vi "C400_module_SR.vi"() -> ()   [LabVIEW 2018]
panel:
  in  "autoconnect":bool=TRUE
  out "Ch1 Position Units":string
  out "Ch1Range":i32
  out "Ch1 Sensor Read":dbl format="%.3f"
  out "Serial Numbers":string[](array[string])
  out "FT_Status":u64(ring) items=["FT_OK", "FT_INVALID_HANDLE", "FT_DEVICE_NOT_FOUND", "FT_DEVICE_NOT_OPENED", "FT_IO_ERROR", "FT_INSUFFICIENT_RESOURCES", "FT_INVALID_PARAMETER", "FT_INVALID_BAUD_RATE", "FT_DEVICE_NOT_OPENED_FOR_ERASE", "FT_DEVICE_NOT_OPENED_FOR_WRITE", "FT_FAILED_TO_WRITE_DEVICE", "FT_EEPROM_READ_FAILED", "FT_EEPROM_WRITE_FAILED", "FT_EEPROM_ERASE_FAILED", "FT_EEPROM_NOT_PRESENT", "FT_EEPROM_NOT_PROGRAMMED", "FT_INVALID_ARGS", "FT_NOT_SUPPORTED", "FT_OTHER_ERROR"]
  in  "Ch1 Position Set":dbl step=50.0 format="%.3f"
  in  "Connect":bool
  in  "Stop VI":bool caption="Stop Button"
  in  "Found piezos":i32(listbox)=-1
  in  "Handle":u64
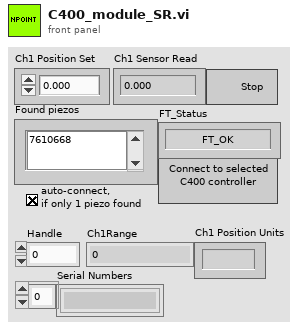
[diagram p1: front panel]
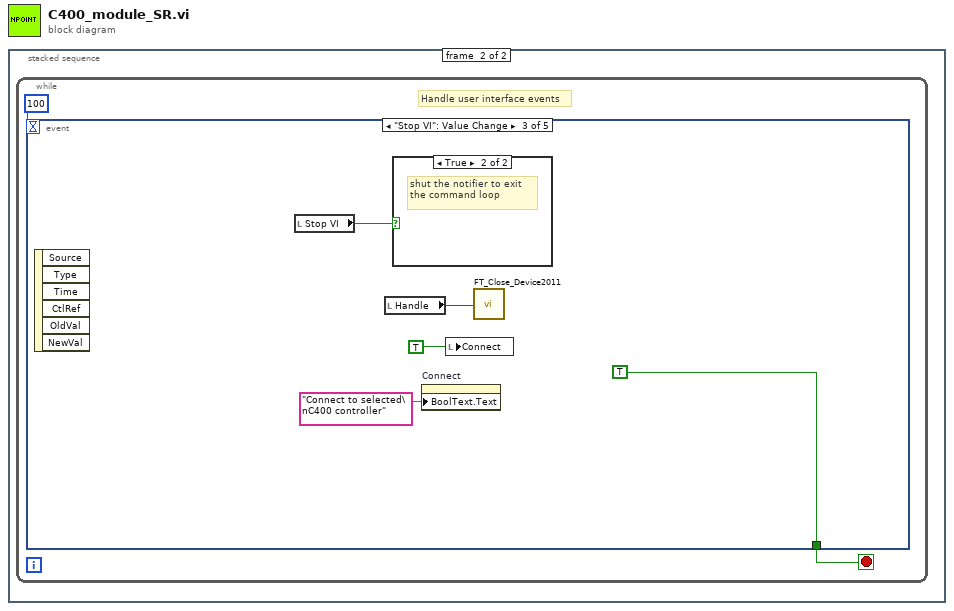
[diagram p0: block diagram]
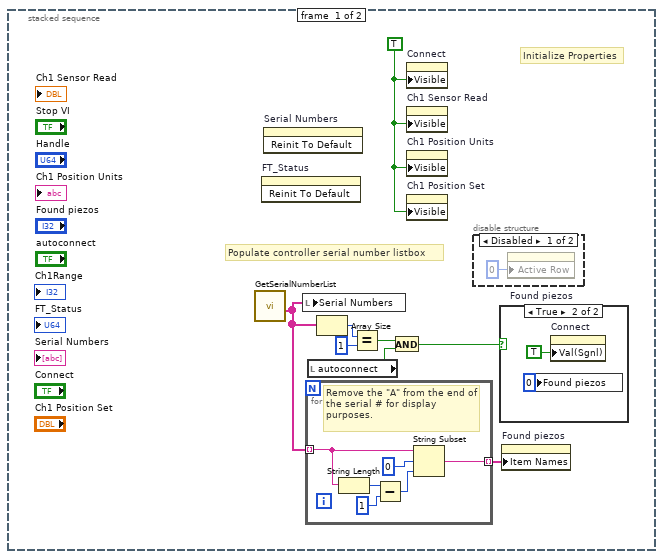
[diagram p2: hidden frame]
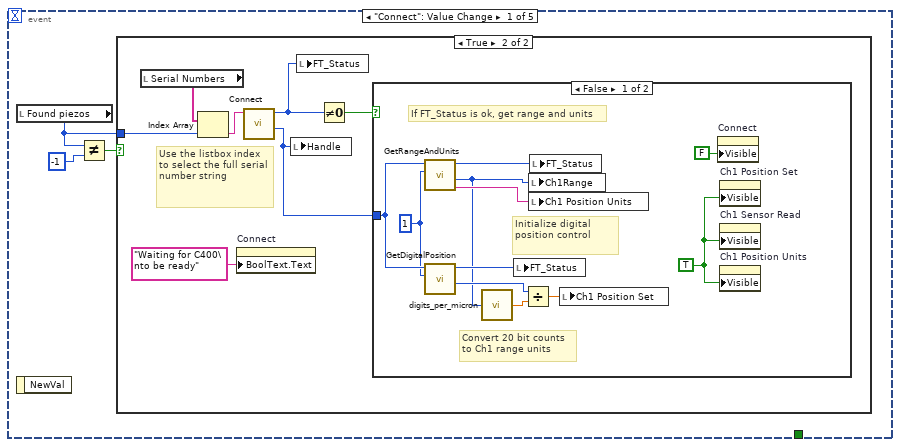
[diagram p5: hidden frame]
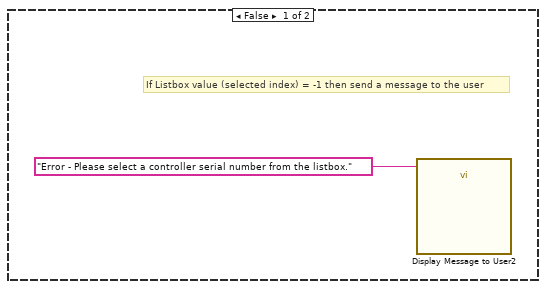
[diagram p6: hidden frame]
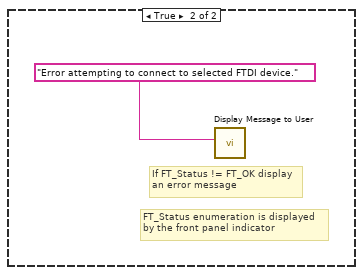
[diagram p7: hidden frame]
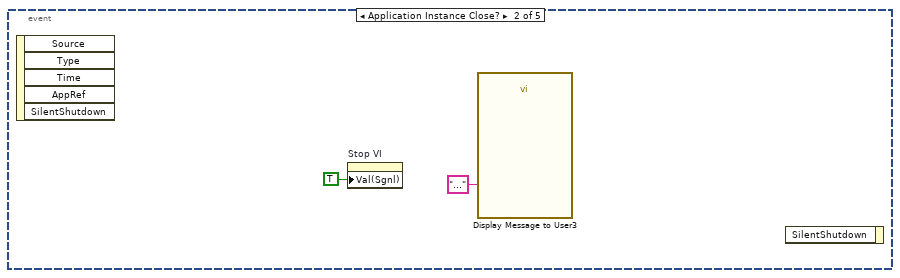
[diagram p8: hidden frame]
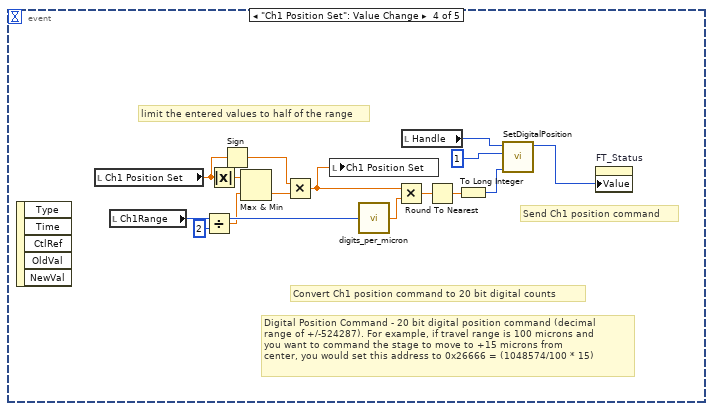
[diagram p10: hidden frame]
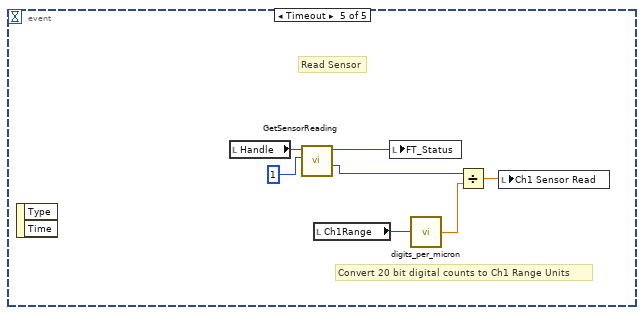
[diagram p11: hidden frame]
diagram:
  n1 = stacked-sequence {
    frame #0 {
      w1 = TRUE ("Visible")
      # "Initialize Properties"
      # "Populate controller serial number listbox"
      n2 = call "GetSerialNumberList.vi"() -> ("C400 Serial Number Array"=w2:string[])  [unwired: 11 in]
      n3 = invoke on="FT_Status" class="Ring (strict)" method="Reinit To Default"() -> ()  [unwired: 3 in, 3 out]
      n4 = invoke on="Serial Numbers" class="Arr (strict)" method="Reinit To Default"() -> ()  [unwired: 3 in, 3 out]
      n5 = local write "Serial Numbers"(w2) -> ()
      n6 = for {
        tunnel: [w13] -> w8 mode=indexing
        tunnel: w2 -> [w12] mode=indexing
        # "Remove the \"A\" from the end of the serial # for display purposes."
        n7 = String Length(string=w12) -> (length=w16:i32)
        n8 = Subtract(x=w16, y=1) -> (x-y=w14:i32)
        n9 = String Subset(string=w12, offset (0)=0, length (rest)=w14) -> (substring=w13:string)
      }
      n10 = local read "autoconnect"() -> (w4:bool)
      n11 = Array Size(array=w2) -> (size(s)=w6:i32)
      n12 = Equal?(x=w6, y=1) -> (x = y?=w3:bool)
      n13 = And(x=w3, y=w4) -> (x .and. y?=w7:bool)
      n14 = property on="Connect" class="Bool (strict)"("Visible"=w1) -> ()  [unwired: 2 in, 2 out]
      n15 = property on="Ch1 Sensor Read" class="DigNum (strict)"("Visible"=w1) -> ()  [unwired: 2 in, 2 out]
      n16 = property on="Ch1 Position Units" class="Str"("Visible"=w1) -> ()  [unwired: 2 in, 2 out]
      n17 = property on="Ch1 Position Set" class="DigNum (strict)"("Visible"=w1) -> ()  [unwired: 2 in, 2 out]
      n18 = disable-structure shown="Disabled" {
        frame Disabled {
          n19 = property on="Found piezos" class="LstBox (strict)"("Active Row"=0 ("Active Row:Active Row Number")) -> ()  [unwired: 2 in, 2 out]
        }
        frame Enabled {
        }
      }
      n20 = case shown="True" w7 {
        frame False {
        }
        frame True {
          n21 = local write "Found piezos"(0 ("Listbox")) -> ()
          n22 = property on="Connect" class="Bool (strict)"("Val(Sgnl)"=TRUE ("Value (Signaling)")) -> ()  [unwired: 2 in, 2 out]
        }
      }
      n23 = property on="Found piezos" class="LstBox (strict)"("Item Names"=w8) -> ()  [unwired: 2 in, 2 out]
    }
    frame #1 {
      n24 = while {
        stop <- w19 stop-if-true
        # "Handle user interface events"
        n25 = event shown="[2] \"Stop VI\": Value Change" {
          selector: _ -> [_ _ _ _ _]
          dyn-events: _ -> [_ _ _ _ _]
          timeout: 100 -> [_ _ _ _ _]
          tunnel: [_ _ TRUE _ _] -> w19
          event "Connect": Value Change {
            n26 = local read "Found piezos"() -> (w20:i32)
            n27 = event-data() -> ()  [unwired: 1 in, 1 out]
            n28 = Not Equal?(x=w20, y=-1) -> (x != y?=w22:bool)
            n29 = case shown="True" w22 {
              tunnel: w20 -> [_ w30]
              frame False {
                # "If Listbox value (selected index) = -1 then send a message to the user"
                n30 = call "Display Message to User2"("Message"="Error - Please select a controller serial number from the listbox.") -> ()  [unwired: 9 in, 2 out]
              }
              frame True {
                # "Use the listbox index to select the full serial number string"
                n31 = local read "Serial Numbers"() -> (w27:string[])
                n32 = Index Array(array=w27, index=w30) -> (element=w28:string)
                n33 = property on="Connect" class="Bool (strict)"("BoolText.Text"="Waiting for C400\nto be ready" ("Boolean Text.Text")) -> ()  [unwired: 2 in, 2 out]
                n34 = call "Connect.vi"("Device Serial Number"=w28) -> ("Handle"=w29:u64, "FT_Status"=w25:u64)  [unwired: 9 in]
                n35 = local write "Handle"(w29) -> ()
                n36 = local write "FT_Status"(w25) -> ()
                n37 = Not Equal To 0?(x=w25) -> (x != 0?=w24:bool)
                n38 = case shown="False" w24 {
                  tunnel: w29 -> [w37 _]
                  frame False {
                    w34 = TRUE ("Visible")
                    w31 = i64 1 ("Controller Channel")
                    # "Convert 20 bit counts\nto Ch1 range units"
                    # "Initialize digital position control"
                    # "If FT_Status is ok, get range and units"
                    n39 = call "GetRangeAndUnits.vi"("Handle"=w37, "Controller Channel"=w31) -> ("FT_Status"=w39:u64, "Range"=w32:i32, "Range Units"=w38:string)  [unwired: 6 in]
                    n40 = call "GetDigitalPosition.vi"("Handle"=w37, "Controller Channel"=w31) -> ("FT_Status"=w35:u64, "Position"=w41:i64)  [unwired: 7 in]
                    n41 = call "digits_per_micron.vi"("Ch1Range"=w32) -> ("digital_per_micron"=w33:dbl)
                    n42 = local write "FT_Status"(w35) -> ()
                    n43 = Divide(x=w41, y=w33) -> (x/y=w36:dbl)
                    n44 = local write "Ch1Range"(w32) -> ()
                    n45 = local write "Ch1 Position Units"(w38) -> ()
                    n46 = local write "FT_Status"(w39) -> ()
                    n47 = local write "Ch1 Position Set"(w36) -> ()
                    n48 = property on="Connect" class="Bool (strict)"("Visible"=FALSE) -> ()  [unwired: 2 in, 2 out]
                    n49 = property on="Ch1 Position Set" class="DigNum (strict)"("Visible"=w34) -> ()  [unwired: 2 in, 2 out]
                    n50 = property on="Ch1 Sensor Read" class="DigNum (strict)"("Visible"=w34) -> ()  [unwired: 2 in, 2 out]
                    n51 = property on="Ch1 Position Units" class="Str"("Visible"=w34) -> ()  [unwired: 2 in, 2 out]
                  }
                  frame True {
                    # "FT_Status enumeration is displayed\nby the front panel indicator"
                    # "If FT_Status != FT_OK display\nan error message"
                    n52 = call "Display Message to User"("Message"="Error attempting to connect to selected FTDI device.") -> ()  [unwired: 9 in, 2 out]
                  }
                }
              }
            }
          }
          event Application Instance Close? {
            n53 = event-data() -> ()  [unwired: 1 in, 5 out]
            n54 = property on="Stop VI" class="Bool (strict)"("Val(Sgnl)"=TRUE ("Value (Signaling)")) -> ()  [unwired: 2 in, 2 out]
            n55 = call "Display Message to User3"("Message"="...") -> ()  [unwired: 9 in, 2 out]
            n56 = event-data() -> ()  [unwired: 2 in, 1 out]
          }
          event "Stop VI": Value Change {
            n57 = event-data() -> ()  [unwired: 1 in, 6 out]
            n58 = local read "Stop VI"() -> (w45:bool)
            n59 = local read "Handle"() -> (w47:u64)
            n60 = case shown="True" w45 {
              frame False {
              }
              frame True {
                # "shut the notifier to exit the command loop"
              }
            }
            n61 = property on="Connect" class="Bool (strict)"("BoolText.Text"="Connect to selected\nC400 controller" ("Boolean Text.Text")) -> ()  [unwired: 2 in, 2 out]
            n62 = local write "Connect"(TRUE ("Visible")) -> ()
            n63 = call "FT_Close_Device2011.vi"("Handle"=w47) -> ()  [unwired: 1 out]
          }
          event "Ch1 Position Set": Value Change {
            # "limit the entered values to half of the range"
            # "Digital Position Command - 20 bit digital position command (decimal\nrange of +/-524287). For example, if travel range is 100 microns and\nyou want to command the stage to move to +15 microns from\ncenter, you would set this address to 0x26666 = (1048574/100 * 15)"
            # "Send Ch1 position command"
            # "Convert Ch1 position command to 20 bit digital counts"
            n64 = event-data() -> ()  [unwired: 1 in, 5 out]
            n65 = local read "Ch1 Position Set"() -> (w53:dbl)
            n66 = local read "Ch1Range"() -> (w57:i32)
            n67 = Divide(x=w57, y=2) -> (x/y=w55:dbl)
            n68 = Absolute Value(x=w53) -> (abs(x)=w54:dbl)
            n69 = Sign(1:w53) -> (0:w51:dbl)
            n70 = Max & Min(x=w54, y=w55) -> (min(x,y)=w52:dbl)  [unwired: 1 out]
            n71 = Multiply(x=w51, y=w52) -> (x*y=w50:dbl)
            n72 = local write "Ch1 Position Set"(w50) -> ()
            n73 = call "digits_per_micron.vi"("Ch1Range"=w57) -> ("digital_per_micron"=w58:dbl)
            n74 = Multiply(x=w50, y=w58) -> (x*y=w62:dbl)
            n75 = local read "Handle"() -> (w59:u64)
            n76 = Round To Nearest(number=w62) -> (nearest integer value=w61:dbl)
            n77 = To Long Integer(number=w61) -> (32bit integer=w60:i32)
            n78 = call "SetDigitalPosition.vi"("Position"=w60, "Controller Channel"=i64 1, "Handle"=w59) -> ("FT_Status"=w63:u64)  [unwired: 8 in]
            n79 = property on="FT_Status" class="Ring (strict)"("Value"=w63) -> ()  [unwired: 2 in, 2 out]
          }
          event Timeout {
            # "Read Sensor"
            # "Convert 20 bit digital counts to Ch1 Range Units"
            n80 = event-data() -> ()  [unwired: 1 in, 2 out]
            n81 = local read "Handle"() -> (w69:u64)
            n82 = call "GetSensorReading.vi"("Handle"=w69, "Controller Channel"=i64 1) -> ("FT_Status"=w70:u64, "Sensor Reading"=w71:i64)  [unwired: 7 in]
            n83 = local read "Ch1Range"() -> (w66:i32)
            n84 = local write "FT_Status"(w70) -> ()
            n85 = call "digits_per_micron.vi"("Ch1Range"=w66) -> ("digital_per_micron"=w67:dbl)
            n86 = Divide(x=w71, y=w67) -> (x/y=w68:dbl)
            n87 = local write "Ch1 Sensor Read"(w68) -> ()
          }
        }
      }
    }
  }
